vi "Init.vi"(8 "error in":errorcluster, 11 "Scope VISA CFG in":refnum<class "Scope VISA CFG.lvclass">) -> (0 "error out":errorcluster, 3 "Scope VISA CFG out":refnum<class "Scope VISA CFG.lvclass">)   [LabVIEW 2023, in "Scope.lvlib" / "Scope VISA.lvlib" / "Scope VISA CFG.lvclass"]
uses:
  Scope VISA CFG.lvclass
  Scope VISA CFG.lvclass/Scope VISA CFG.ctl
  Configuration Base/Configuration Base.lvclass
  2b7bcb15-04f4-4e40-91e9-05d441e86d6e.vi
  <vilib>/ErrorRing/Error Ring.xnode
  <vilib>/Utility/error.llb/Error Cluster From Error Code.vi
panel:
  out "obsolete data":string
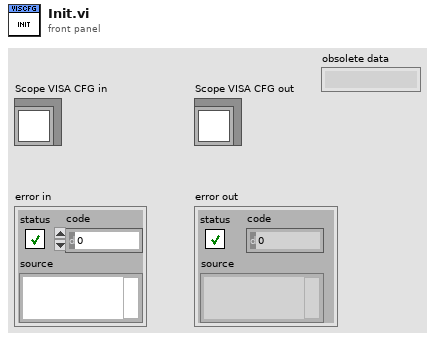
[diagram p1: front panel]
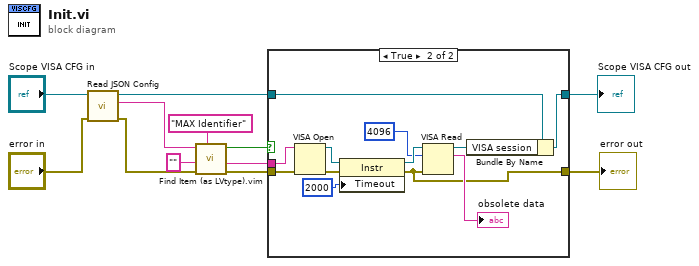
[diagram p0: block diagram]
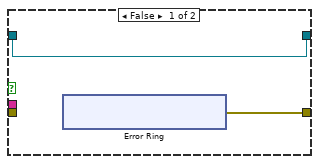
[diagram p2: hidden frame]
diagram:
  n1 = call "Read JSON Config.vi"("error in"="error in", "object in"="Scope VISA CFG in") -> ("error out"=w9:errorcluster, "<JSON>Config"=w7:string, "object out"=w2:refnum<class "Scope VISA CFG.lvclass">)  [unwired: 7 in]
  n2 = call "Find Item (as LVtype).vim"("$Path or Item Name"="MAX Identifier", "error in (no error)"=w9, "Data Type and Default Value"="", "JSON"=w7) -> ("error out"=w8:errorcluster, "Data"=w4:string, "Found"=w3:bool)  [unwired: 4 in, 1 out]
  n3 = case shown="True" w3 {
    tunnel: [w13 w20] -> w12
    tunnel: w8 -> [_ w31]
    tunnel: w4 -> [_ w30]
    tunnel: w2 -> [w14 w29]
    tunnel: [w14 w28] -> w1
    frame False {
      n4 = xnode "Error Ring"() -> ("error out"=w13:errorcluster)
    }
    frame True {
      n5 = VISA Open(error in (no error)=w31, VISA resource name=w30) -> (VISA resource name=w26:refnum<visa-resource-name>, error out=w25:errorcluster)  [unwired: 3 in]
      n6 = property class="Instr"(reference=w26, error in=w25, "Timeout"=u32 2000 ("General Settings:Timeout Value")) -> (reference out=w24:refnum<visa-resource-name>, error out=w20:errorcluster)
      n7 = VISA Read(VISA resource name=w24, byte count=u32 4096, error in (no error)=w20) -> (VISA resource name out=w23:refnum<visa-resource-name>, read buffer=→"obsolete data":string)  [unwired: 2 out]
      n8 = Bundle By Name(cluster=w29, "VISA session"=w23) -> (w28:refnum<class "Scope VISA CFG.lvclass">)
    }
  }
  "error out" <- w12
  "Scope VISA CFG out" <- w1
